vi "Get Data from Modbus.vi"(8 "error in (no error)":errorcluster, 10 "Data":u16[](array[numeric]), 11 "GUI in":refnum<class "GUI.lvclass">) -> (0 "error out":errorcluster, 3 "GUI out":refnum<class "GUI.lvclass">)   [LabVIEW 2020, in "GUI.lvlib" / "GUI.lvclass"]
uses:
  GUI.lvclass
  GUI.lvclass/GUI.ctl
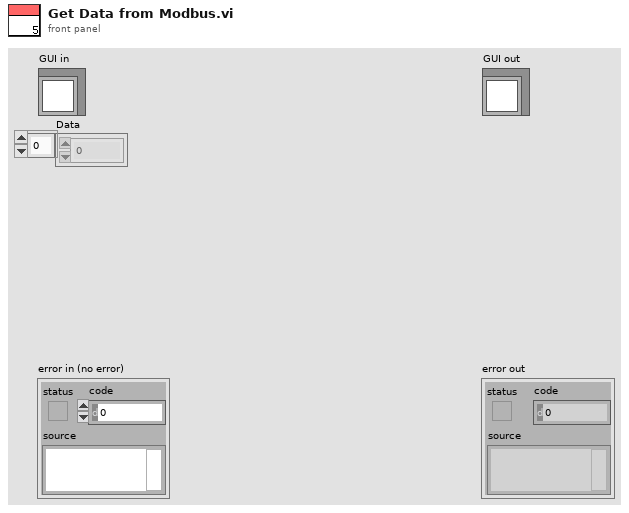
[diagram p1: front panel]
types:
  T1 = cluster{"LDO":i32, "LAI":i32, "Control":i32, "Connect":i32}
  T2 = cluster{"Boolean 9":bool, "Boolean 7":bool, "Boolean 5":bool, "Boolean 3":bool, "Boolean 1":bool, "Boolean 10":bool, "Boolean 8":bool, "Boolean 6":bool, "Boolean 4":bool, "Boolean 2":bool}
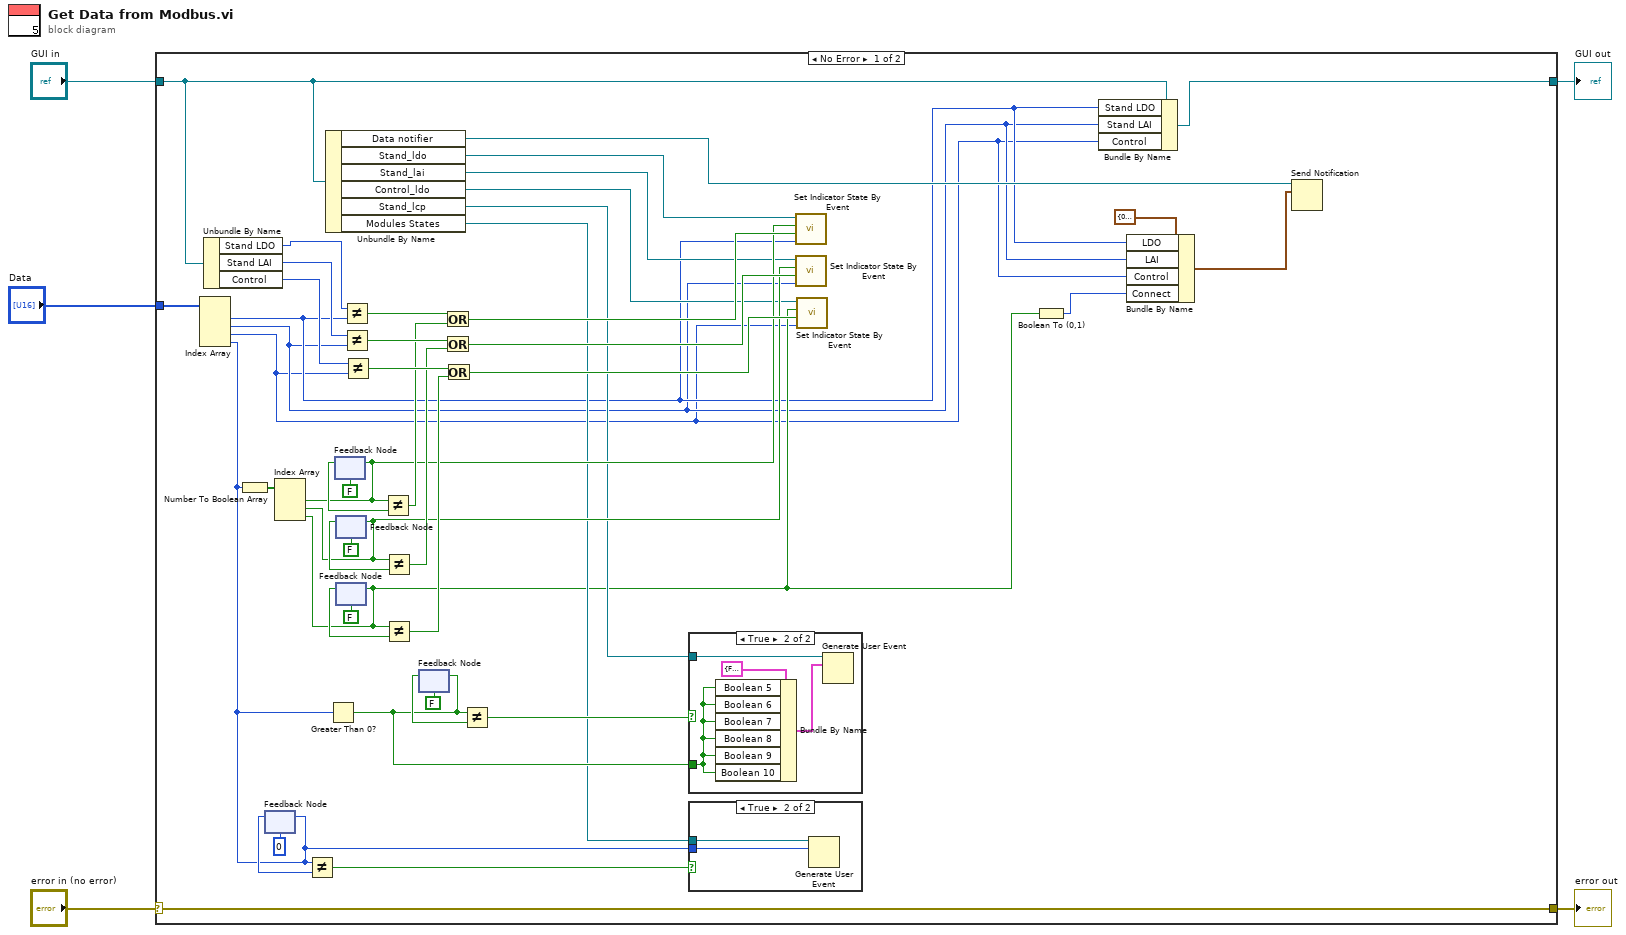
[diagram p0: block diagram]
diagram:
  n1 = case shown="No Error" "error in (no error)" {
    selector: "error in (no error)" -> [w51 w59]
    tunnel: [w51 w59] -> w4
    tunnel: [w47 w58] -> w2
    tunnel: "GUI in" -> [w48 w58]
    tunnel: "Data" -> [w50 _]
    frame No Error {
      n2 = Index Array(array=w50) -> (element #1=w8:u16, element #2=w7:u16, element #3=w6:u16, element #4=w19:u16)  [unwired: 4 in]
      n3 = Unbundle By Name(w48) -> ("Stand LDO"=w13:u16, "Stand LAI"=w12:u16, "Control"=w11:u16)
      n4 = Number To Boolean Array(number=w19) -> (Boolean array=w46:bool[])
      n5 = feedback #1(u16 0 ("Numeric")) -> (w20:u16)
      n6 = feedback-in #1(w19) -> ()
      n7 = Index Array(array=w46) -> (element #1=w30:bool, element #2=w29:bool, element #3=w16:bool)  [unwired: 3 in]
      n8 = Not Equal?(x=w19, y=w20) -> (x != y?=w17:bool)
      n9 = Unbundle By Name(w48) -> ("Data notifier"=w15:refnum<notifier>, "Stand_ldo"=w49:refnum<user-event>, "Stand_lai"=w28:refnum<user-event>, "Control_ldo"=w27:refnum<user-event>, "Stand_lcp"=w22:refnum<user-event>, "Modules States"=w18:refnum<user-event>)
      n10 = Greater Than 0?(x=w19) -> (x > 0?=w23:bool)
      n11 = feedback-in #2(w30) -> ()
      n12 = feedback #2(FALSE) -> (w44:bool)
      n13 = feedback #3(FALSE) -> (w41:bool)
      n14 = feedback-in #3(w29) -> ()
      n15 = feedback #4(FALSE) -> (w40:bool)
      n16 = feedback-in #4(w16) -> ()
      n17 = Not Equal?(x=w13, y=w8) -> (x != y?=w39:bool)
      n18 = Not Equal?(x=w12, y=w7) -> (x != y?=w38:bool)
      n19 = Not Equal?(x=w11, y=w6) -> (x != y?=w37:bool)
      n20 = Not Equal?(x=w30, y=w44) -> (x != y?=w36:bool)
      n21 = Not Equal?(x=w29, y=w41) -> (x != y?=w35:bool)
      n22 = Not Equal?(x=w16, y=w40) -> (x != y?=w34:bool)
      n23 = feedback #5(FALSE) -> (w25:bool)
      n24 = feedback-in #5(w23) -> ()
      n25 = Or(x=w39, y=w36) -> (x .or. y?=w33:bool)
      n26 = Or(x=w38, y=w35) -> (x .or. y?=w32:bool)
      n27 = Or(x=w37, y=w34) -> (x .or. y?=w31:bool)
      n28 = Not Equal?(x=w23, y=w25) -> (x != y?=w24:bool)
      n29 = case shown="True" w24 {
        tunnel: w23 -> [_ w54]
        tunnel: w22 -> [_ w57]
        frame False {
        }
        frame True {
          n30 = Bundle By Name(cluster=T2 {"Boolean 9"=FALSE, "Boolean 7"=FALSE, "Boolean 5"=FALSE, "Boolean 3"=FALSE, "Boolean 1"=FALSE, "Boolean 10"=FALSE, "Boolean 8"=FALSE, "Boolean 6"=FALSE, "Boolean 4"=FALSE, "Boolean 2"=FALSE} ("event data"), "Boolean 5"=w54, "Boolean 6"=w54, "Boolean 7"=w54, "Boolean 8"=w54, "Boolean 9"=w54, "Boolean 10"=w54) -> (w55:T2)
          n31 = Generate User Event(user event=w57, event data cluster=w55) -> ()  [unwired: 2 in, 2 out]
        }
      }
      n32 = case shown="True" w17 {
        tunnel: w19 -> [_ w52]
        tunnel: w18 -> [_ w53]
        frame False {
        }
        frame True {
          n33 = Generate User Event(user event=w53, event data cluster=w52) -> ()  [unwired: 2 in, 2 out]
        }
      }
      n34 = call "Set Indicator State By Event.vi"("Value"=w8, "New Value?"=w33, "No error"=w30, "Module Indicator Event"=w49) -> ()  [unwired: 8 in]
      n35 = call "Set Indicator State By Event.vi"("Value"=w7, "New Value?"=w32, "No error"=w29, "Module Indicator Event"=w28) -> ()  [unwired: 8 in]
      n36 = call "Set Indicator State By Event.vi"("Value"=w6, "New Value?"=w31, "No error"=w16, "Module Indicator Event"=w27) -> ()  [unwired: 8 in]
      n37 = Boolean To (0,1)(Boolean=w16) -> (0, 1=w10:i16)
      n38 = Bundle By Name(cluster=w48, "Stand LDO"=w8, "Stand LAI"=w7, "Control"=w6) -> (w47:refnum<class "GUI.lvclass">)
      n39 = Bundle By Name(cluster=T1 {"LDO"=0, "LAI"=0, "Control"=0, "Connect"=0} ("data value"), "LDO"=w8, "LAI"=w7, "Control"=w6, "Connect"=w10) -> (w9:T1)
      n40 = Send Notification(notification=w9, notifier=w15) -> ()  [unwired: 1 in, 2 out]
    }
    frame Error {
    }
  }
  "error out" <- w4
  "GUI out" <- w2
